vi "Configure Partial IO.vi"(0 "VISA resource name":refnum<visa-resource-name>, 1 "Boundary (0)":i32, 5 "Channel (0001)":string="0001", 7 "Enable Partial Expand (Off)":bool, 9 "Expand (50%)":i32=50, 11 "error in (no error)":errorcluster) -> (4 "VISA resource name out":refnum<visa-resource-name>, 6 "Channel":string, 15 "error out":errorcluster)   [LabVIEW 2020, in "Yokogawa GX Series.lvlib"]
doc: "Sets the partial expanded display on I/O channel.\n\nCommand: SPartialIO\n\nNote: This VI does nothing when the instrument is GM10."
uses:
  <instrlib>/Yokogawa GX Series/Yokogawa GX Series.lvlib
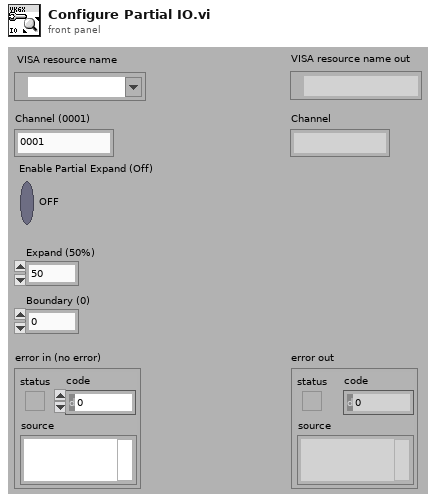
[diagram p1: front panel]
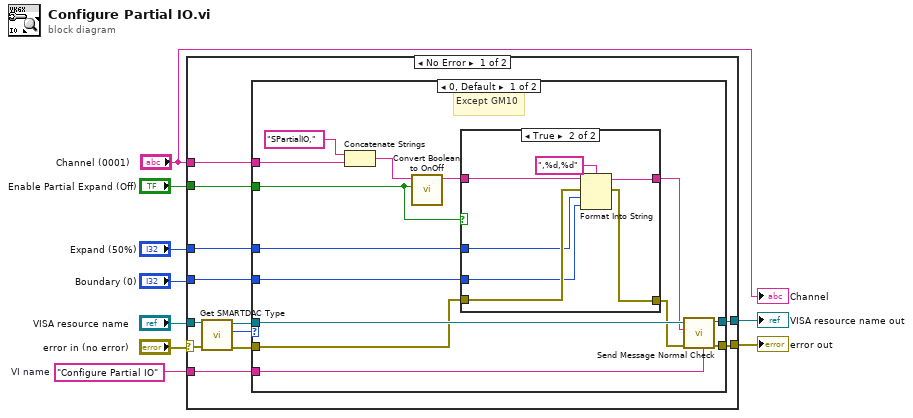
[diagram p0: block diagram]
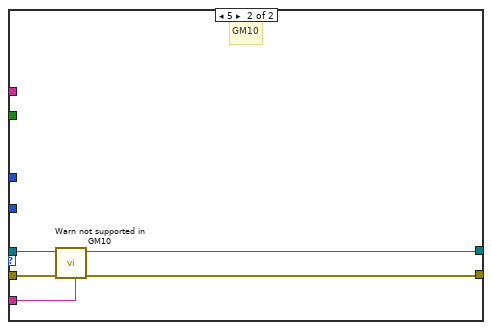
[diagram p3: hidden frame]
diagram:
  w8 = "Configure Partial IO"  # VI name
  n1 = case shown="No Error" "error in (no error)" {
    selector: "error in (no error)" -> [w13 w50]
    tunnel: "VISA resource name" -> [w14 w51]
    tunnel: w8 -> [w21 _]
    tunnel: [w20 w51] -> w7
    tunnel: [w19 w50] -> w6
    tunnel: "Channel (0001)" -> [w18 _]
    tunnel: "Enable Partial Expand (Off)" -> [w17 _]
    tunnel: "Expand (50%)" -> [w16 _]
    tunnel: "Boundary (0)" -> [w15 _]
    frame No Error {
      n2 = call <instrlib>:"Get SMARTDAC Type.vi"("error in (no error)"=w13, "VISA resource name"=w14) -> ("error out"=w11:errorcluster, "SMARTDAC+ Type"=w10:u16, "VISA resource name out"=w12:refnum<visa-resource-name>)  [unwired: 7 in]
      n3 = case shown="0, Default" w10 {
        tunnel: w12 -> [w35 w49]
        tunnel: w21 -> [w34 w45]
        tunnel: [w33 w47] -> w20
        tunnel: [w32 w46] -> w19
        tunnel: w11 -> [w22 w48]
        tunnel: w18 -> [w24 _]
        tunnel: w17 -> [w31 _]
        tunnel: w16 -> [w30 _]
        tunnel: w15 -> [w29 _]
        frame 0, Default {
          # "Except GM10"
          n4 = Concatenate Strings("SPartialIO,", w24) -> (w23:string)
          n5 = call <instrlib>:"Convert Boolean to OnOff.vi"("On/Off"=w31, "Initial String (\"\")"=w23) -> ("Resulting String"=w28:string)  [unwired: 9 in]
          n6 = case shown="True" w31 {
            tunnel: w30 -> [_ w41]
            tunnel: w29 -> [_ w39]
            tunnel: w28 -> [w37 w44]
            tunnel: [w37 w38] -> w27
            tunnel: w22 -> [w36 w43]
            tunnel: [w36 w40] -> w26
            frame False {
            }
            frame True {
              n7 = Format Into String(format string=",%d,%d", initial string=w44, error in=w43, w41, w39) -> (resulting string=w38:string, error out=w40:errorcluster)
            }
          }
          n8 = call <instrlib>:"Send Message Normal Check.vi"("Source (\"\")"=w34, "error in (no error)"=w26, "Send Message (\"\")"=w27, "VISA resource name"=w35) -> ("error out"=w32:errorcluster, "VISA resource name out"=w33:refnum<visa-resource-name>)  [unwired: 1 in, 5 out]
        }
        frame 5 {
          # "GM10"
          n9 = call <instrlib>:"Warn not supported in GM10.vi"("Source (\"\")"=w45, "error in (no error)"=w48, "VISA resource name"=w49) -> ("error out"=w46:errorcluster, "VISA resource name out"=w47:refnum<visa-resource-name>)  [unwired: 7 in]
        }
      }
    }
    frame Error {
    }
  }
  "error out" <- w6
  "VISA resource name out" <- w7
  "Channel" <- "Channel (0001)"
